vi "Disabled.vi"(7 "Robot Mode":T2, 10 "Match Info":T1={"Autonomous Elapsed Seconds"=0.0, "TeleOp Elapsed Seconds"=0.0, "Disabled Elapsed Seconds"=0.0, "Visited Autonomous"=FALSE, "Visited TeleOp"=FALSE, "Visited Disabled"=FALSE, "Autonomous Settings"={"Autonomous Style"=enum."Independent", "VI Refnum"=refnum}}, 11 "Call Context":T3) -> ()   [LabVIEW 2018]
doc: "This VI is called each time a disabled packet is received from the DS. It is often used to prepare for the next robot mode, to calibrate sensors, etc."
uses:
  <vilib>/Rock Robotics/WPI/DriverStation/WPI_DriverStationDerivedRobotMode.ctl
  <vilib>/Rock Robotics/WPI/DriverStation/WPI_DriverStationRobotMode2.ctl
  <vilib>/Rock Robotics/WPI/DriverStation/WPI_DriverStationMatch Info.ctl
  Subsytems/Drive/Drive_Notifier.ctl
  Subsytems/Drive/Drive_Control_Type.ctl
  Subsytems/Climb/Climb_Notifier.ctl
  Subsytems/Climb/Climb_Control_Type.ctl
  Subsytems/Elevator/Elevator_Notifier.ctl
  Subsytems/Elevator/Elevator_Control_Type.ctl
  Subsytems/Elevator/Elevator_Enum_States.ctl
  Subsytems/Intake_Joint/Intake_Joint_Notifier.ctl
  Subsytems/Intake_Joint/Intake_Joint_Control_Type.ctl
  Subsytems/Intake_Joint/Intake_Joint_Enum_States.ctl
  Subsytems/Intake_Ball/Intake_Ball_Notifier.ctl
  Subsytems/Intake_Ball/Intake_Ball_Control_Type.ctl
  Subsytems/Intake_Disc/Intake_Disc_Notifier.ctl
  Subsytems/Intake_Disc/Intake_Disc_Control_Type.ctl
  <vilib>/Rock Robotics/WPI/Solenoid/WPI_SolenoidValue.ctl
  Global_Variables/Elevator_Globals.vi
  Global_Variables/Climb_Globals.vi
  Global_Variables/Drive_Globals.vi
  Global_Variables/LED_Globals.vi
  Global_Variables/Autonomous_Globals.vi
  Global_Variables/Intake_Joint_Globals.vi
  Global_Variables/Refnum_Names.vi
  <vilib>/Rock Robotics/WPI/Utilities/WPI_GetSetVariantRefNum.vi
  Global_Variables/Intake_Ball_Globals.vi
  Global_Variables/Intake_Disc_Globals.vi
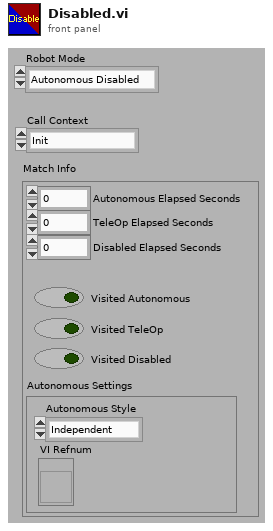
[diagram p1: front panel]
types:
  T1 = typedef "WPI_DriverStationMatch Info.ctl" = cluster{"Autonomous Elapsed Seconds":dbl, "TeleOp Elapsed Seconds":dbl, "Disabled Elapsed Seconds":dbl, "Visited Autonomous":bool, "Visited TeleOp":bool, "Visited Disabled":bool, "Autonomous Settings":cluster{"Autonomous Style":enum16{"Iterative", "Independent"}, "VI Refnum":refnum<vi>}}
  T2 = typedef "WPI_DriverStationRobotMode2.ctl" = enum16{"Autonomous Disabled", "Autonomous Enabled", "Teleop Disabled", "Teleop Enabled", "Disconnected", "Finish", "Test Disabled", "Test Enabled", "Emergency Stopped"}
  T3 = typedef "WPI_DriverStationDerivedRobotMode.ctl" = enum16{"Init", "Execute", "Stop"}
  T4 = typedef "Intake_Disc_Notifier.ctl" = cluster{"Intake_Disc_Control_Type":T5, "Manual_Disc_Toggle":bool, "Disc_Toggle":bool, "Disc_Toggle_State":bool, "Manual_Press_Toggle":bool, "Disc_Press_State":bool, "Press_Toggle":bool, "Press_Pnuematic":T6, "Disc_Pnuematic":T6, "Disc_Notifier":refnum<notifier>, "Step":i32}
  T5 = typedef "Intake_Disc_Control_Type.ctl" = enum16{"No_Op", "Manual_Disc_Toggle", "Disc_Toggle", "Manual_Press_Toggle", "Press_Toggle", "Acquire_Hatch", "Retract"}
  T6 = typedef "WPI_SolenoidValue.ctl" = enum16{"Off", "On", "Forward", "Reverse"}
  T7 = typedef "Intake_Ball_Notifier.ctl" = cluster{"Intake_Ball_Control_Type":T8, "Manual_In":bool, "Manual_Out":bool, "Ball_In":bool, "Ball_Out":bool, "Parameter_One":dbl, "Parameter_Two":dbl, "Parameter_Three":dbl, "Step":i32, "Ball_Notifier":refnum<notifier>}
  T8 = typedef "Intake_Ball_Control_Type.ctl" = enum16{"No_Op", "Manual_In", "Manual_Out", "In_Sensor_Stop", "Out_Teleop", "Out", "Stall"}
  T9 = typedef "Intake_Joint_Notifier.ctl" = cluster{"Intake_Joint_Control_Type":T10, "Manual_Joint_Up":bool, "Manual_Joint_Down":bool, "Low_Rocket":bool, "Mid_Rocket":bool, "High_Rocket":bool, "Cargo_Ship":bool, "Hatch_Floor":bool, "Cargo_Floor":bool, "HP_Hatch":bool, "HP_Cargo":bool, "Depot_Cargo":bool, "Stow":bool, "Intake_Mode":bool, "Set Position":T11, "Parameter_One":dbl, "Parameter_Two":dbl, "Parameter_Three":dbl, "Step":i32, "Joint_Notifier":refnum<notifier>}
  T10 = typedef "Intake_Joint_Control_Type.ctl" = enum16{"No_Op", "Manual_Joint_Up", "Manual_Joint_Down", "Manual_Position_Control", "Position_Control", "Position"}
  T11 = typedef "Intake_Joint_Enum_States.ctl" = enum16{"Current_Position", "High_Rocket_Hatch_Panel_Floor", "High_Rocket_Hatch_Panel", "Mid_Rocket_Hatch_Panel_Floor", "Mid_Rocket_Hatch_Panel", "Low_Rocket_Hatch_Panel", "Cargo_Ship_Hatch_Panel", "Loading_Station_Hatch_Panel", "Ground_Pickup_Hatch_Panel", "High_Rocket_Cargo", "Mid_Rocket_Cargo", "Low_Rocket_Cargo", "Cargo_Ship_Cargo", "Loading_Station_Cargo", "Ground_Pickup_Cargo", "Depot_Pickup_Cargo", "Stow_Cargo", "Get_Hatch"}
  T12 = typedef "Elevator_Notifier.ctl" = cluster{"Elevator_Control_Type":T13, "Shift":bool, "Brake":bool, "Manual_Lift_Up":bool, "Manual_Lift_Down":bool, "Climb_Advance":bool, "Climb_Reverse":bool, "Low_Rocket":bool, "Mid_Rocket":bool, "High_Rocket":bool, "Cargo_Ship":bool, "Hatch_Floor":bool, "Cargo_Floor":bool, "HP_Hatch":bool, "HP_Cargo":bool, "Depot_Cargo":bool, "Stow":bool, "Set_Position":T14, "Intake_Mode":bool, "Climb_Distance":dbl, "Level_Two":bool, "Parameter_One":dbl, "Parameter_Two":dbl, "Parameter_Three":dbl, "Step":i32, "Elevator_Notifier":refnum<notifier>, "Brake_State":bool, "Shift_State":bool}
  T13 = typedef "Elevator_Control_Type.ctl" = enum16{"No_Op", "Shift", "Brake", "Manual_Elevator_Up", "Manual_Elevator_Down", "Manual_Climb_Up", "Manual_Climb_Down", "Manual_Position_Control", "Elevator_Retract", "Elevator_Extend", "Brake_In_Climb", "Position_Control", "Position", "Shift_Climb"}
  T14 = typedef "Elevator_Enum_States.ctl" = enum16{"Current_Position", "High_Rocket_Hatch_Panel_Floor", "High_Rocket_Hatch_Panel", "Mid_Rocket_Hatch_Panel_Floor", "Mid_Rocket_Hatch_Panel", "Low_Rocket_Hatch_Panel", "Cargo_Ship_Hatch_Panel", "Loading_Station_Hatch_Panel", "Ground_Pickup_Hatch_Panel", "High_Rocket_Cargo", "Mid_Rocket_Cargo", "Low_Rocket_Cargo", "Cargo_Ship_Cargo", "Loading_Station_Cargo", "Ground_Pickup_Cargo", "Depot_Pickup_Cargo", "Descend_Off_Platform", "Stow_Cargo"}
  T15 = typedef "Climb_Notifier.ctl" = cluster{"Climb_Control_Type":T16, "Brake":bool, "Manual_Climb_Up":bool, "Manual_Drive_Forward":bool, "Manual_Drive_Backward":bool, "Manual_Climb_Down":bool, "Climb_Advance":bool, "Climb_Reverse":bool, "Parameter_One":dbl, "Parameter_Two":dbl, "Parameter_Three":dbl, "Step":i32, "Climb_Notifier":refnum<notifier>, "Climb_Distance":dbl, "Level_Two":bool, "Brake_State":bool, "Toggle_Servo":bool}
  T16 = typedef "Climb_Control_Type.ctl" = enum16{"No_Op", "Brake", "Manual_Climb_Up", "Manual_Climb_Down", "Manual_Drive_Forward", "Manual_Drive_Backward", "Back_Wheels_Forward", "Lift_Retract", "Lift_Extend", "Extend_to_Second_Level", "Spin"}
  T17 = typedef "Drive_Notifier.ctl" = cluster{"Drive Control List":T18, "Front/Back":dbl, "Left/Right":dbl, "Turn":dbl, "Test_Joy_Y":dbl, "Test_Joy_X":dbl, "Set Wheel Encoder Positions":bool, "Robotcentric":bool, "Reset Gyro":bool, "Rotate Front Right":bool, "Rotate Front Left":bool, "Rotate Back Right":bool, "Rotate Back Left":bool, "Write_Encoder_Positions":bool, "Climb_Advance":bool, "Parameter_One":dbl, "Parameter_Two":dbl, "Parameter_Three":dbl, "Parameter_Four":dbl, "Drive_Notifier":refnum<notifier>, "Step":i32, "Climb_Reverse":bool, "Auto_Target":bool}
  T18 = typedef "Drive_Control_Type.ctl" = enum16{"No_Op", "Write_FL_Position", "Write_FR_Position", "Write_BL_Position", "Write_BR_Position", "Set_Encoder_Positions", "Fieldcentric_PercentVBus", "Fieldcentric", "Robotcentric", "Reset_Gyro", "FR_Wheel", "FL_Wheel", "BR_Wheel", "BL_Wheel", "Drive_Onto_Platform", "Manual_Wheel_Control", "Distance", "Turn_To_Heading", "Turn_To_Target", "Drive_To_Target", "Zero", "Auto_Target", "Drive_Over_Platform", "Heading_Lock", "Time"}
  T19 = typedef "WPI_JoystickDevRef.ctl" = cluster{"Device":T20}
  T20 = typedef "WPI_JoystickDeviceEnum.ctl" = enum16{"USB 0", "USB 1", "USB 2", "USB 3", "USB 4", "USB 5"}
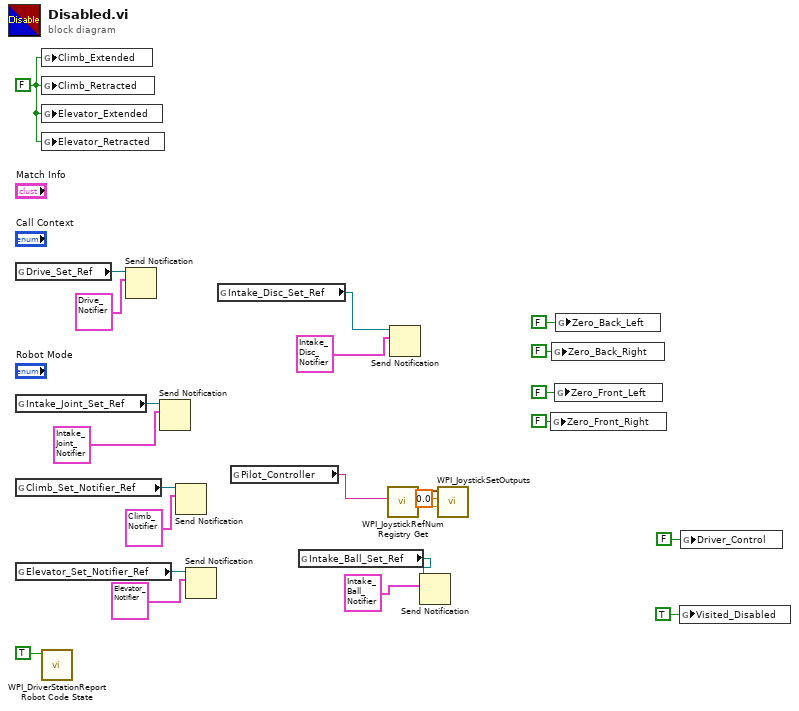
[diagram p0: block diagram]
diagram:
  w12 = sgl 0.0 ("Left Rumble")
  w18 = FALSE
  n1 = global read "Drive_Globals.vi" "Drive_Set_Ref"() -> (w22:refnum<notifier>)
  n2 = global read "Intake_Joint_Globals.vi" "Intake_Joint_Set_Ref"() -> (w17:refnum<notifier>)
  n3 = global read "Climb_Globals.vi" "Climb_Set_Notifier_Ref"() -> (w19:refnum<notifier>)
  n4 = global read "Elevator_Globals.vi" "Elevator_Set_Notifier_Ref"() -> (w16:refnum<notifier>)
  n5 = global write "Climb_Globals.vi" "Climb_Extended"(w18) -> ()
  n6 = global write "Climb_Globals.vi" "Climb_Retracted"(w18) -> ()
  n7 = global write "Elevator_Globals.vi" "Elevator_Extended"(w18) -> ()
  n8 = global write "Elevator_Globals.vi" "Elevator_Retracted"(w18) -> ()
  n9 = call <vilib>:"WPI_DriverStationReport Robot Code State.vi"("Disabled"=TRUE ("Autonomous")) -> ()  [unwired: 10 in, 1 out]
  n10 = Send Notification(notification=T17 {"Drive Control List"=enum."No_Op", "Front/Back"=0.0, "Left/Right"=0.0, "Turn"=0.0, "Test_Joy_Y"=0.0, "Test_Joy_X"=0.0, "Set Wheel Encoder Positions"=FALSE, "Robotcentric"=FALSE, "Reset Gyro"=FALSE, "Rotate Front Right"=FALSE, "Rotate Front Left"=FALSE, "Rotate Back Right"=FALSE, "Rotate Back Left"=FALSE, "Write_Encoder_Positions"=FALSE, "Climb_Advance"=FALSE, "Parameter_One"=0.0, "Parameter_Two"=0.0, "Parameter_Three"=0.0, "Parameter_Four"=0.0, "Drive_Notifier"=refnum, "Step"=0, "Climb_Reverse"=FALSE, "Auto_Target"=FALSE} ("Drive Notifier"), notifier=w22) -> ()  [unwired: 1 in, 2 out]
  n11 = Send Notification(notification=T9 {"Intake_Joint_Control_Type"=enum."No_Op", "Manual_Joint_Up"=FALSE, "Manual_Joint_Down"=FALSE, "Low_Rocket"=FALSE, "Mid_Rocket"=FALSE, "High_Rocket"=FALSE, "Cargo_Ship"=FALSE, "Hatch_Floor"=FALSE, "Cargo_Floor"=FALSE, "HP_Hatch"=FALSE, "HP_Cargo"=FALSE, "Depot_Cargo"=FALSE, "Stow"=FALSE, "Intake_Mode"=FALSE, "Set Position"=enum."Current_Position", "Parameter_One"=0.0, "Parameter_Two"=0.0, "Parameter_Three"=0.0, "Step"=0, "Joint_Notifier"=refnum} ("Intake_Joint_Notifier"), notifier=w17) -> ()  [unwired: 1 in, 2 out]
  n12 = Send Notification(notification=T15 {"Climb_Control_Type"=enum."No_Op", "Brake"=FALSE, "Manual_Climb_Up"=FALSE, "Manual_Drive_Forward"=FALSE, "Manual_Drive_Backward"=FALSE, "Manual_Climb_Down"=FALSE, "Climb_Advance"=FALSE, "Climb_Reverse"=FALSE, "Parameter_One"=0.0, "Parameter_Two"=0.0, "Parameter_Three"=0.0, "Step"=0, "Climb_Notifier"=refnum, "Climb_Distance"=0.0, "Level_Two"=FALSE, "Brake_State"=FALSE, "Toggle_Servo"=FALSE} ("Climb_Notifier"), notifier=w19) -> ()  [unwired: 1 in, 2 out]
  n13 = Send Notification(notification=T12 {"Elevator_Control_Type"=enum."No_Op", "Shift"=FALSE, "Brake"=FALSE, "Manual_Lift_Up"=FALSE, "Manual_Lift_Down"=FALSE, "Climb_Advance"=FALSE, "Climb_Reverse"=FALSE, "Low_Rocket"=FALSE, "Mid_Rocket"=FALSE, "High_Rocket"=FALSE, "Cargo_Ship"=FALSE, "Hatch_Floor"=FALSE, "Cargo_Floor"=FALSE, "HP_Hatch"=FALSE, "HP_Cargo"=FALSE, "Depot_Cargo"=FALSE, "Stow"=FALSE, "Set_Position"=enum."Current_Position", "Intake_Mode"=FALSE, "Climb_Distance"=0.0, "Level_Two"=FALSE, "Parameter_One"=0.0, "Parameter_Two"=0.0, "Parameter_Three"=0.0, "Step"=0, "Elevator_Notifier"=refnum, "Brake_State"=FALSE, "Shift_State"=FALSE} ("Elevator_Notifier"), notifier=w16) -> ()  [unwired: 1 in, 2 out]
  n14 = global read "Intake_Disc_Globals.vi" "Intake_Disc_Set_Ref"() -> (w3:refnum<notifier>)
  n15 = global read "Refnum_Names.vi" "Pilot_Controller"() -> (w11:string)
  n16 = global read "Intake_Ball_Globals.vi" "Intake_Ball_Set_Ref"() -> (w9:refnum<notifier>)
  n17 = call <vilib>:"WPI_JoystickRefNum Registry Get.vi"("refnum name"=w11) -> ("JoystickDevRef"=w13:T19)  [unwired: 9 in, 1 out]
  n18 = Send Notification(notification=T4 {"Intake_Disc_Control_Type"=enum."No_Op", "Manual_Disc_Toggle"=FALSE, "Disc_Toggle"=FALSE, "Disc_Toggle_State"=FALSE, "Manual_Press_Toggle"=FALSE, "Disc_Press_State"=FALSE, "Press_Toggle"=FALSE, "Press_Pnuematic"=enum."Forward", "Disc_Pnuematic"=enum."Forward", "Disc_Notifier"=refnum, "Step"=0} ("Intake_Disc_Notifier"), notifier=w3) -> ()  [unwired: 1 in, 2 out]
  n19 = Send Notification(notification=T7 {"Intake_Ball_Control_Type"=enum."No_Op", "Manual_In"=FALSE, "Manual_Out"=FALSE, "Ball_In"=FALSE, "Ball_Out"=FALSE, "Parameter_One"=0.0, "Parameter_Two"=0.0, "Parameter_Three"=0.0, "Step"=0, "Ball_Notifier"=refnum} ("Intake_Ball_Notifier"), notifier=w9) -> ()  [unwired: 1 in, 2 out]
  n20 = call <vilib>:"WPI_JoystickSetOutputs.vi"("Right Rumble"=w12, "Left Rumble"=w12, "JoystickDevRef"=w13) -> ()  [unwired: 7 in, 2 out]
  n21 = global write "Drive_Globals.vi" "Zero_Front_Right"(FALSE ("Zero_Back_Left")) -> ()
  n22 = global write "Drive_Globals.vi" "Zero_Back_Right"(FALSE ("Zero_Back_Left")) -> ()
  n23 = global write "Drive_Globals.vi" "Zero_Front_Left"(FALSE ("Zero_Back_Left")) -> ()
  n24 = global write "Drive_Globals.vi" "Zero_Back_Left"(FALSE ("Zero_Back_Left")) -> ()
  n25 = global write "LED_Globals.vi" "Visited_Disabled"(TRUE ("Visited_Disabled")) -> ()
  n26 = global write "Autonomous_Globals.vi" "Driver_Control"(FALSE ("Driver_Control")) -> ()
